vi "06 - Extensions.vi"() -> ()   [LabVIEW 2015]
uses:
  Libraries/LibSDL2 Wrapper/Controls/Rectangle.ctl
  Libraries/LibSDL2 Wrapper/Controls/Init Flags.ctl
  Libraries/LibSDL2 Wrapper/Controls/Surface.ctl
  <vilib>/Utility/importsl/GetValueByPointer/datatype.ctl
  Libraries/LibSDL2 Wrapper/Controls/NULL.ctl
  <vilib>/Utility/importsl/GetValueByPointer/GetValueByPointer.xnode
  Libraries/LibSDL2 Wrapper/LibSDL2.lvlib
  Libraries/SDL2 Utility/SDL2 Utility.lvlib
  Libraries/LibSDL2_Image Wrapper/LibSDL2_Image.lvlib
panel:
  in  "Scale":bool
  in  "Destination Rectangle":T1={"x"=-123, "y"=-114, "Width"=553, "Height"=415}
  in  "Source Rectangle":T1={"x"=0, "y"=0, "Width"=622, "Height"=495}
  out "Error":string
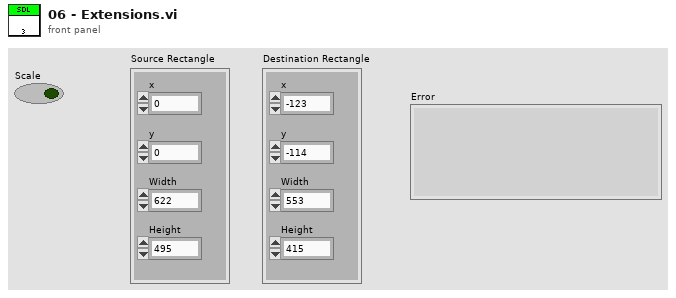
[diagram p1: front panel]
types:
  T1 = typedef "LibSDL2.lvlib/Rectangle.ctl" = cluster{"x":i32, "y":i32, "Width":i32, "Height":i32}
  T2 = enum32{"pack1", "pack2", "pack4", "pack8", "pack16"}
  T3 = typedef "LibSDL2.lvlib/Surface.ctl" = cluster{"Flags":u32, "Pixel Format Pointer":u32, "Width":i32, "Height":i32, "Pitch":i32, "Pixels Pointer":u32, "User Data Pointer":u32, "Locked":i32, "Lock Data Pointer":u32, "Clip Rectangle":T1, "Blitmap Pointer":u32, "Ref Count":i32}
  T4 = typedef "LibSDL2.lvlib/Init Flags.ctl" = u32
  T5 = typedef "LibSDL2.lvlib/NULL.ctl" = enum32{"NULL"}
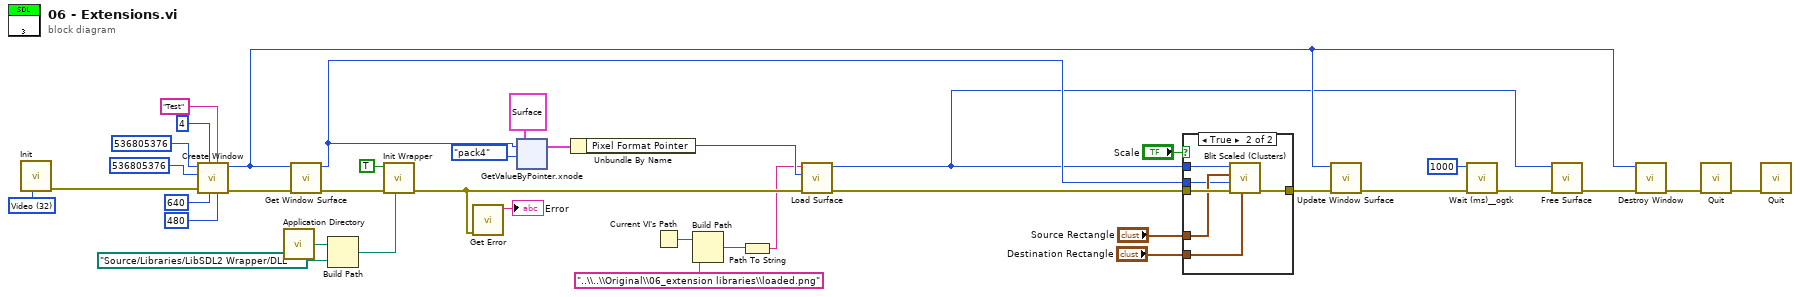
[diagram p0: block diagram]
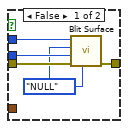
[diagram p2: hidden frame]
diagram:
  w38 = T4 32 items=["Timer"=1, "Audio"=16, "Video"=32, "Joystick"=512, "Haptic"=4096, "Game Controller"=8192, "Events"=16384, "No Parachute"=1048576, "Everything"=17244689] ("Init Flags")
  n1 = call "Init.vi"("Flags"=w38) -> ("error out"=w32:errorcluster)  [unwired: 9 in, 1 out]
  n2 = call "Create Window.vi"("Height"=480, "Title"="Test", "Width"=640, "Flags"=u32 4, "error in"=w32, "Position y"=u32 536805376 ("Flags"), "Position x"=u32 536805376 ("Flags")) -> ("error out"=w28:errorcluster, "Window Pointer"=w22:u32)  [unwired: 3 in]
  n3 = call <vilib>:"Application Directory.vi"() -> ("Application Directory"=w8:path)
  n4 = call "Get Window Surface.vi"("error in"=w28, "Window Pointer"=w22) -> ("error out"=w16:errorcluster, "Surface Pointer"=w21:u32)  [unwired: 8 in]
  n5 = Build Path(base path=w8, name or relative path=path "Source/Libraries/LibSDL2 Wrapper/DLL" ("DLL Directory")) -> (appended path=w6:path)
  n6 = call "Init Wrapper.vi"("DLL Directory"=w6, "error in"=w16, "PNG (F)"=TRUE ("PNG")) -> ("error out"=w13:errorcluster)  [unwired: 7 in, 1 out]
  n7 = call "Get Error.vi"("error in"=w13) -> ("Error"=→"Error":string)  [unwired: 9 in, 1 out]
  n8 = xnode "GetValueByPointer.xnode"("Pointer"=w21, "InputType"=T3 {"Flags"=0, "Pixel Format Pointer"=0, "Width"=0, "Height"=0, "Pitch"=0, "Pixels Pointer"=0, "User Data Pointer"=0, "Locked"=0, "Lock Data Pointer"=0, "Clip Rectangle"={"x"=0, "y"=0, "Width"=0, "Height"=0}, "Blitmap Pointer"=0, "Ref Count"=0} ("Surface"), "PackType"=T2."pack4") -> ("Output"=w23:T3)  [unwired: 1 in, 1 out]
  n9 = Unbundle By Name(w23) -> ("Pixel Format Pointer"=w18:u32)
  n10 = Current VI's Path() -> (path=w4:path)
  n11 = Build Path(base path=w4, name or relative path="..\\..\\Original\\06_extension libraries\\loaded.png" ("File")) -> (appended path=w3:path)
  n12 = Path To String(path=w3) -> (string=w1:string)
  n13 = call "Load Surface.vi"("error in"=w13, "Pixel Format Pointer"=w18, "File"=w1) -> ("error out"=w19:errorcluster, "Optimised Surface Pointer"=w17:u32)  [unwired: 7 in]
  n14 = case shown="True" "Scale" {
    tunnel: w21 -> [w43 w45]
    tunnel: w17 -> [w42 w47]
    tunnel: w19 -> [w41 w49]
    tunnel: [w40 w48] -> w12
    tunnel: "Source Rectangle" -> [_ w46]
    tunnel: "Destination Rectangle" -> [_ w44]
    frame False {
      w39 = NULL."NULL" ("Null")
      n15 = call "Blit Surface.vi"("Destination Rectangle Pointer"=w39, "error in"=w41, "Destination Surface Pointer"=w43, "Source Rectangle Pointer"=w39, "Source Surface Pointer"=w42) -> ("error out"=w40:errorcluster)  [unwired: 5 in, 1 out]
    }
    frame True {
      n16 = call "Blit Scaled (Clusters).vi"("Destination Rectangle"=w44, "error in"=w49, "Destination Surface Pointer"=w45, "Source Rectangle"=w46, "Source Surface Pointer"=w47) -> ("error out"=w48:errorcluster)  [unwired: 5 in, 1 out]
    }
  }
  n17 = call "Update Window Surface.vi"("error in"=w12, "Window Pointer"=w22) -> ("error out"=w20:errorcluster)  [unwired: 9 in]
  n18 = call <userlib>:"Wait (ms)__ogtk.vi"("error in (no error)"=w20, "milliseconds to wait"=u32 1000) -> ("error out"=w27:errorcluster)  [unwired: 8 in, 1 out]
  n19 = call "Free Surface.vi"("error in"=w27, "Surface Pointer"=w17) -> ("error out"=w26:errorcluster)  [unwired: 9 in]
  n20 = call "Destroy Window.vi"("error in"=w26, "Window Pointer"=w22) -> ("error out"=w15:errorcluster)  [unwired: 9 in]
  n21 = call "Quit.vi"("error in"=w15) -> ("error out"=w14:errorcluster)  [unwired: 10 in]
  n22 = call "Quit.vi"("error in"=w14) -> ()  [unwired: 10 in, 1 out]
